vi "Periodic Tasks.vi"(8 "error in":errorcluster) -> ()   [LabVIEW 2018]
doc: "This VI runs in parallel to other robot code. It can contain as many user-defined periodic loops as you need. These can carry out PID or other sorts of timed response."
uses:
  <vilib>/Rock Robotics/SystemInterfaces/AI/FPGA_AIChannel.ctl
  <vilib>/Rock Robotics/Network Tables/NT Write Number.vi
  <vilib>/Rock Robotics/Network Tables/NT Write Boolean.vi
  Robot Global Data.vi
  <vilib>/Rock Robotics/Network Tables/NT Write Variant.vi
  <vilib>/Rock Robotics/WPI/Power/WPI_Power Get 5Volt Rail Voltage and Current.vi
  ADIS16448 IMU/ADIS16448_IMU.lvlib
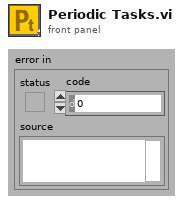
[diagram p1: front panel]
types:
  T1 = typedef "FPGA_AIChannel.ctl" = enum8{"AI 0", "AI 1", "AI 2", "AI 3", "AI MXP 0", "AI MXP 1", "AI MXP 2", "AI MXP 3", "Invalid"}
  T2 = typedef "WPI_AnalogChannelDevRef.ctl" = cluster{"DevStatus":errorcluster, "Analog Channel":T1}
  T3 = typedef "Command Status Info.ctl" = cluster{"Name":string, "Status":T4, "notifier out":T5}
  T4 = typedef "Completion Status.ctl" = enum16{"Successful", "Aborted", "Incomplete"}
  T5 = typedef "Completion Notifier.ctl" = refnum<notifier>
  T6 = typedef "NetComm_ControlWord.ctl" = cluster{"Enabled":bool, "Autonomous":bool, "Test":bool, "E-Stop":bool, "FMS Attached":bool, "DS Attached":bool}
  T7 = typedef "ADIS16448_IMU.lvlib/ADI_IMU_ADIS16448_IMUDevRef.ctl" = cluster{"DevStatus":errorcluster, "Handle":i32, "SPI Bus":T8, "Device Found":bool, "Device Ready":bool, "Yaw Axis":enum16{"X", "Y", "Z"}, "AHRS Algorithm":enum16{"Complementary", "Madgwick"}, "Serial":u16, "Lot ID 2":u16, "Lot ID 1":u16, "Bytes Per Sample":u16, "Calibrate On Open?":bool}
  T8 = typedef "spi_bus.ctl" = enum16{"SPI On-Board, CS0", "SPI On-Board, CS1", "SPI On-Board, CS2", "SPI On-Board, CS3", "SPI MXP", "Invalid"}
  T9 = typedef "WPI_DriverStationRobotMode2.ctl" = enum16{"Autonomous Disabled", "Autonomous Enabled", "Teleop Disabled", "Teleop Enabled", "Disconnected", "Finish", "Test Disabled", "Test Enabled", "Emergency Stopped"}
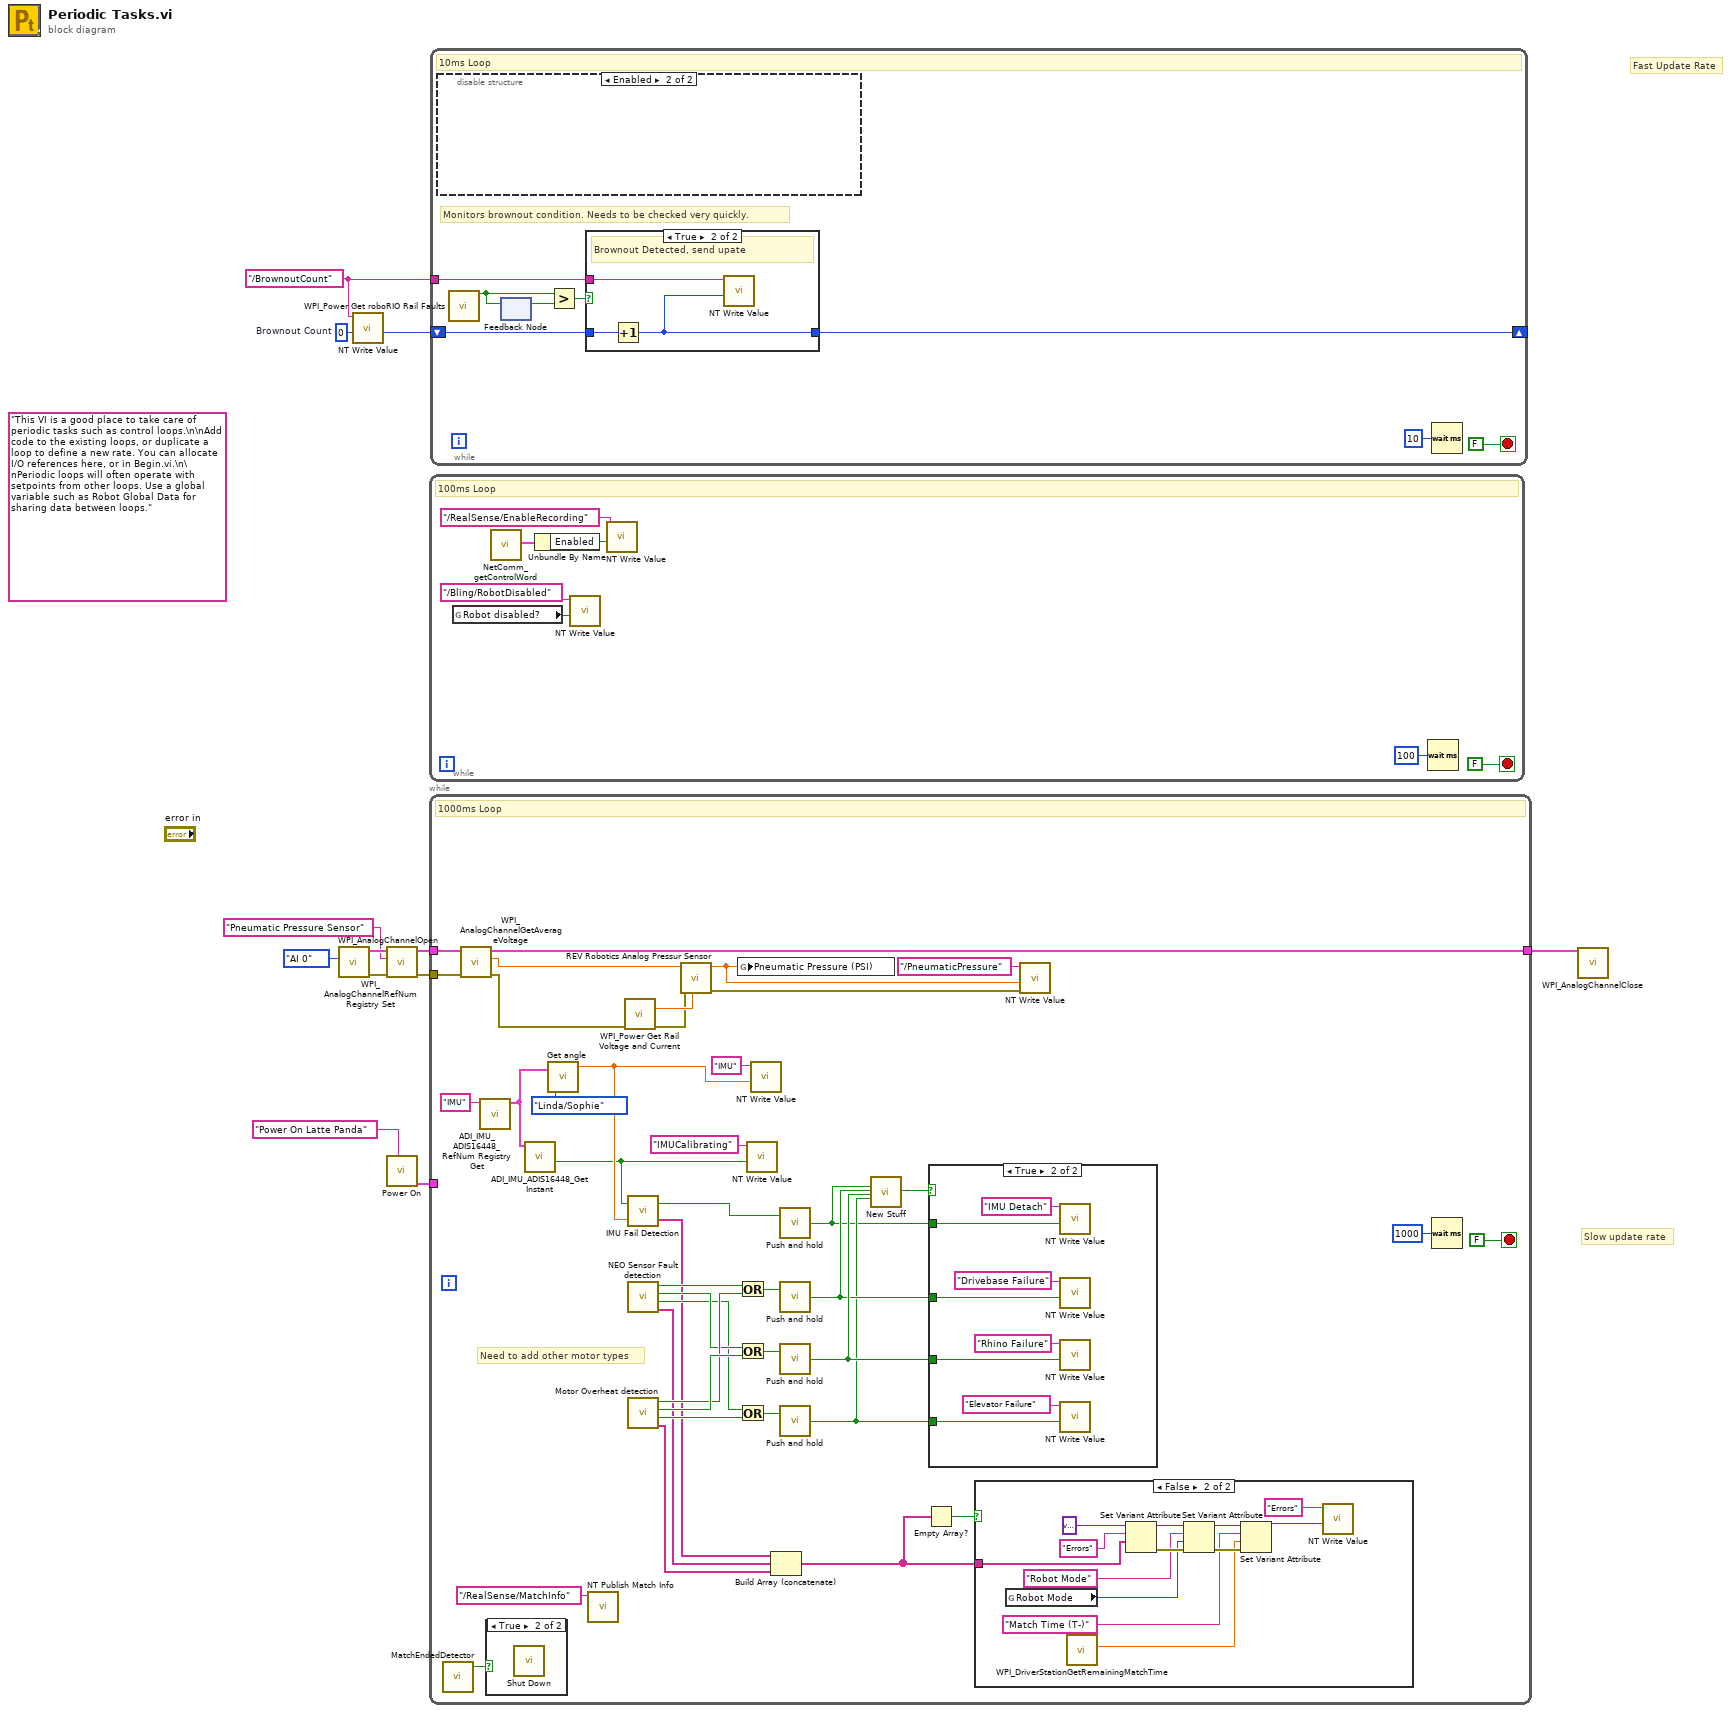
[diagram p0: block diagram]
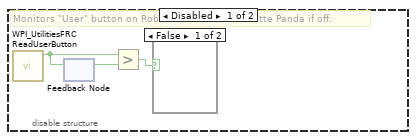
[diagram p5: hidden frame]
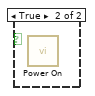
[diagram p6: hidden frame]
diagram:
  w10 = "/BrownoutCount" ("Name")
  w11 = 0  # Brownout Count
  (unwired) "This VI is a good place to take care of periodic tasks such as control loops.\n\nAdd code to the existing loops, or duplicate a loop to define a new rate. You can allocate I/O references here, or in Begin.vi.\n\nPeriodic loops will often operate with setpoints from other loops. Use a global variable such as Robot Global Data for sharing data between loops."
  # "Slow update rate"
  # "Fast Update Rate"
  n1 = call <vilib>:"WPI_AnalogChannelOpen.vi"("Analog Channel"=FPGA_AIChannel."AI 0") -> ("error out"=w4:errorcluster, "AIDeviceRef"=w3:T2)  [unwired: 9 in]
  n2 = call-poly <vilib>:"NT Write Value.vi"("Numeric"=w11, "Name"=w10) -> ()  [unwired: 9 in, 1 out]
  n3 = call <vilib>:"WPI_AnalogChannelRefNum Registry Set.vi"("error in (no error)"=w4, "refnum name"="Pneumatic Pressure Sensor", "AIDeviceRef"=w3) -> ("error out"=w8:errorcluster, "AIDeviceRef"=w9:T2)  [unwired: 7 in]
  n4 = call "Power On.vi"("Description"="Power On Latte Panda") -> ("Command Info Out"=w6:T3)  [unwired: 10 in]
  n5 = while {
    stop <- FALSE stop-if-true
    # "100ms Loop"
    n6 = global read "Robot Global Data.vi" "Robot disabled?"() -> (w18:bool)
    n7 = call <vilib>:"NetComm_getControlWord.vi"() -> ("Control Word"=w15:T6)  [unwired: 10 in, 1 out]
    n8 = Unbundle By Name(w15) -> ("Enabled"=w16:bool)
    n9 = call-poly <vilib>:"NT Write Value.vi"("Boolean"=w18, "Name"="/Bling/RobotDisabled") -> ()  [unwired: 9 in, 1 out]
    n10 = call-poly <vilib>:"NT Write Value.vi"("Boolean"=w16, "Name"="/RealSense/EnableRecording") -> ()  [unwired: 9 in, 1 out]
    n11 = Wait (ms)(milliseconds to wait=u32 100) -> ()  [unwired: 1 out]
  }
  n12 = while {
    tunnel: w9 -> [w57]
    tunnel: w8 -> [w58]
    tunnel: [w56] -> w7
    tunnel: w6 -> [_]
    stop <- FALSE stop-if-true
    # "Need to add other motor types"
    # "1000ms Loop"
    n13 = call "MatchEndedDetector.vi"() -> ("Match Ended"=w55:bool)  [unwired: 10 in, 1 out]
    n14 = call <vilib>:"WPI_AnalogChannelGetAverageVoltage.vi"("error in (no error)"=w58, "AIDeviceRef"=w57) -> ("error out"=w35:errorcluster, "Voltage"=w37:dbl, "AIDeviceRef"=w56:T2)  [unwired: 7 in]
    n15 = call "ADI_IMU_ADIS16448_RefNum Registry Get.vi"("refnum name"="IMU") -> ("ADI IMU DevRef"=w49:T7)  [unwired: 9 in, 1 out]
    n16 = case shown="True" w55 {
      frame False {
      }
      frame True {
        n17 = call "Shut Down.vi"() -> ()  [unwired: 11 in, 1 out]
      }
    }
    n18 = call "ADI_IMU_ADIS16448_Get Instant.vi"("ADI IMU DevRef"=w49) -> ("Sensor Ready Out"=w19:bool)  [unwired: 7 in, 3 out]
    n19 = call "Get angle.vi"("ADI IMU DevRef Out"=w49, "Robot"=enum16{"Linda/Sophie", "Mule"}."Linda/Sophie") -> ("Out"=w21:dbl)  [unwired: 2 out]
    n20 = call "NT Publish Match Info.vi"("NT Variable Name"="/RealSense/MatchInfo" ("Name")) -> ()  [unwired: 9 in, 2 out]
    n21 = call-poly <vilib>:"WPI_Power Get Rail Voltage and Current.vi"("error in"=w35) -> ("5 volt rail voltage (V)"=w36:dbl, "error out"=w34:errorcluster)  [unwired: 12 in, 1 out]
    n22 = call "IMU Fail Detection.vi"("IMU Value"=w21, "Boolean"=w19) -> ("Array"=w25:string[], "IMU Error?"=w20:bool)
    n23 = call "NEO Sensor Fault detection.vi"() -> ("Array"=w24:string[], "Cascade Sensor"=w38:bool, "Rhino Sensors"=w39:bool, "Drivebase Sensors"=w40:bool)
    n24 = call "Motor Overheat detection.vi"() -> ("Array"=w23:string[], "Cascade Sensor"=w43:bool, "Rhino Sensors"=w42:bool, "Drivebase Sensors"=w41:bool)
    n25 = call "REV Robotics Analog Pressur Sensor.vi"("Vcc (V)"=w36, "error in (no error)"=w34, "Vout (V)"=w37) -> ("error out"=w33:errorcluster, "Pressure (PSI)"=w32:dbl)  [unwired: 7 in]
    n26 = global write "Robot Global Data.vi" "Pneumatic Pressure (PSI)"(w32) -> ()
    n27 = Or(x=w40, y=w41) -> (x .or. y?=w44:bool)
    n28 = Or(x=w39, y=w42) -> (x .or. y?=w45:bool)
    n29 = Or(x=w38, y=w43) -> (x .or. y?=w46:bool)
    n30 = call-poly <vilib>:"NT Write Value.vi"("Boolean"=w19, "Name"="IMUCalibrating") -> ()  [unwired: 9 in, 1 out]
    n31 = call-poly <vilib>:"NT Write Value.vi"("Numeric"=w21, "Name"="IMU") -> ()  [unwired: 9 in, 1 out]
    n32 = Build Array (concatenate)(w25, w24, w23) -> (w22:string[])
    n33 = call "Push and hold.vi"("Input"=w20) -> ("Output"=w27:bool)  [unwired: 1 in]
    n34 = call "Push and hold.vi"("Input"=w44) -> ("Output"=w29:bool)  [unwired: 1 in]
    n35 = call "Push and hold.vi"("Input"=w45) -> ("Output"=w47:bool)  [unwired: 1 in]
    n36 = call "Push and hold.vi"("Input"=w46) -> ("Output"=w28:bool)  [unwired: 1 in]
    n37 = call "New Stuff.vi"("Variant 4"=w27, "Variant 3"=w29, "Variant 16"=w47, "Variant 15"=w28) -> ("x != y?"=w48:bool)  [unwired: 23 in]
    n38 = Empty Array?(array=w22) -> (empty?=w26:bool)
    n39 = case shown="True" w48 {
      tunnel: w29 -> [_ w77]
      tunnel: w47 -> [_ w76]
      tunnel: w28 -> [_ w75]
      tunnel: w27 -> [_ w73]
      frame False {
      }
      frame True {
        n40 = call-poly <vilib>:"NT Write Value.vi"("Boolean"=w73, "Name"="IMU Detach") -> ()  [unwired: 9 in, 1 out]
        n41 = call-poly <vilib>:"NT Write Value.vi"("Boolean"=w77, "Name"="Drivebase Failure") -> ()  [unwired: 9 in, 1 out]
        n42 = call-poly <vilib>:"NT Write Value.vi"("Boolean"=w76, "Name"="Rhino Failure") -> ()  [unwired: 9 in, 1 out]
        n43 = call-poly <vilib>:"NT Write Value.vi"("Boolean"=w75, "Name"="Elevator Failure") -> ()  [unwired: 9 in, 1 out]
      }
    }
    n44 = case shown="False" w26 {
      tunnel: w22 -> [_ w60]
      frame True {
      }
      frame False {
        n45 = global read "Robot Global Data.vi" "Robot Mode"() -> (w68:T9)
        n46 = call <vilib>:"WPI_DriverStationGetRemainingMatchTime.vi"() -> ("Match Time(s)"=w63:sgl)  [unwired: 10 in, 1 out]
        n47 = Set Variant Attribute(Variant=variant, name="Errors", value=w60) -> (Variant out=w69:variant, error out=w70:errorcluster)  [unwired: 1 in, 1 out]
        n48 = Set Variant Attribute(Variant=w69, name="Robot Mode", value=w68, error in=w70) -> (Variant out=w65:variant, error out=w66:errorcluster)  [unwired: 1 out]
        n49 = Set Variant Attribute(Variant=w65, name="Match Time (T-)", value=w63, error in=w66) -> (Variant out=w62:variant)  [unwired: 2 out]
        n50 = call-poly <vilib>:"NT Write Value.vi"("Variant"=w62, "Name"="Errors") -> ()  [unwired: 9 in, 1 out]
      }
    }
    n51 = call-poly <vilib>:"NT Write Value.vi"("error in"=w33, "Numeric"=w32, "Name"="/PneumaticPressure") -> ()  [unwired: 8 in, 1 out]
    n52 = Wait (ms)(milliseconds to wait=u32 1000) -> ()  [unwired: 1 out]
  }
  n53 = while {
    shift-right: [w84] -> _
    shift-left: w11 -> [w83]
    tunnel: w10 -> [w82]
    stop <- FALSE stop-if-true
    # "Monitors brownout condition. Needs to be checked very quickly."
    # "10ms Loop"
    n54 = disable-structure shown="Enabled" {
      frame Disabled {
        # "Monitors \"User\" button on RoboRIO and turns on Latte Panda if off."
        n55 = call <vilib>:"WPI_UtilitiesFRC ReadUserButton.vi"() -> ("User Button"=w90:bool)  [unwired: 10 in, 1 out]
        n56 = feedback #1() -> (w91:bool)  [unwired: 1 in]
        n57 = feedback-in #1(w90) -> ()
        n58 = Greater?(x=w90, y=w91) -> (0:w89:bool)
        n59 = case shown="False" w89 {
          frame False {
          }
          frame True {
            n60 = call "Power On.vi"() -> ()  [unwired: 11 in, 1 out]
          }
        }
      }
      frame Enabled {
      }
    }
    n61 = call <vilib>:"WPI_Power Get roboRIO Rail Faults.vi"() -> ("Input Voltage Brown Out"=w87:bool)  [unwired: 10 in, 5 out]
    n62 = feedback-in #2(w87) -> ()
    n63 = feedback #2() -> (w86:bool)  [unwired: 1 in]
    n64 = Greater?(x=w87, y=w86) -> (0:w85:bool)
    n65 = case shown="True" w85 {
      tunnel: w83 -> [w92 w95]
      tunnel: [w92 w94] -> w84
      tunnel: w82 -> [_ w93]
      frame False {
        # "No brown out"
      }
      frame True {
        # "Brownout Detected, send upate"
        n66 = Increment(x=w95) -> (x+1=w94:i32)
        n67 = call-poly <vilib>:"NT Write Value.vi"("Numeric"=w94, "Name"=w93) -> ()  [unwired: 9 in, 1 out]
      }
    }
    n68 = Wait (ms)(milliseconds to wait=u32 10) -> ()  [unwired: 1 out]
  }
  n69 = call <vilib>:"WPI_AnalogChannelClose.vi"("AIDeviceRef"=w7) -> ()  [unwired: 10 in, 1 out]
